vi "Read Configuration.vi"(0 "Config File Path":path, 5 "Scalar Or Vector":string="Scalar", 9 "Fixture Or Cal":string="Fixture", 11 "Error in (no error)":errorcluster) -> (4 "Path Groups out":refnum<class "Path Group.lvclass">[](array[class]), 6 "Path Count":i32, 15 "Error out":errorcluster)   [LabVIEW 2023, in "RFCalAndFixtureCharact.Common.lvlib"]
uses:
  RFCalAndFixtureCharact.Common.lvlib
  Base Classes/Path Group/Path Group.lvclass
  <vilib>/Utility/file.llb/Read Delimited Spreadsheet (string).vi
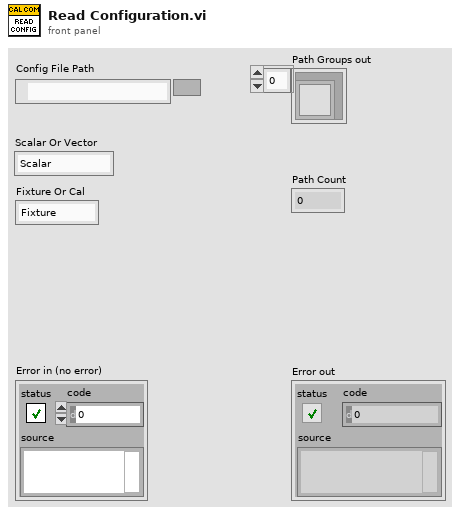
[diagram p1: front panel]
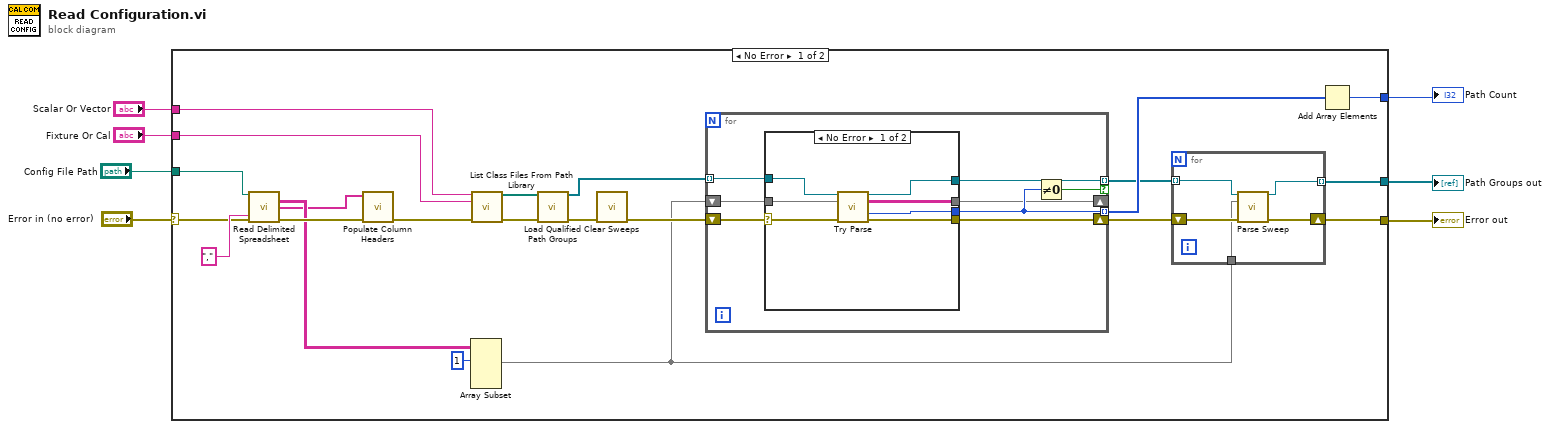
[diagram p0: block diagram]
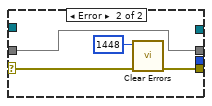
[diagram p2: hidden frame]
diagram:
  n1 = case shown="No Error" "Error in (no error)" {
    selector: "Error in (no error)" -> [w20 w54]
    tunnel: [w8 w54] -> w6
    tunnel: [w27 _] -> w5
    tunnel: "Config File Path" -> [w21 _]
    tunnel: [w10 _] -> w3
    tunnel: "Fixture Or Cal" -> [w17 _]
    tunnel: "Scalar Or Vector" -> [w16 _]
    frame No Error {
      n2 = call-poly <vilib>:"Read Delimited Spreadsheet.vi"("file path (dialog if empty)"=w21, "error in (no error)"=w20, "delimiter (\\t)"="," ("delimiter (\\t)")) -> ("all rows"=w24:string[][], "first row"=w22:string[], "error out"=w25:errorcluster)  [unwired: 7 in, 3 out]
      n3 = call "Populate Column Headers.vi"("error in (no error)"=w25, "Column Headers"=w22) -> ("error out"=w15:errorcluster)  [unwired: 9 in]
      n4 = Array Subset(array=w24, index (row)=1 ("index")) -> (w9:string[][])  [unwired: 3 in]
      n5 = call "List Class Files From Path Library.vi"("Specified Folder Name"=w16, "Fixture Or Cal"=w17, "Error in"=w15) -> ("Class Files"=w18:path[], "Error out"=w19:errorcluster)  [unwired: 11 in]
      n6 = call "Load Qualified Path Groups.vi"("Class Files"=w18, "error in"=w19) -> ("Path Groups out"=w29:refnum<class "Path Group.lvclass">[], "error out"=w14:errorcluster)  [unwired: 12 in]
      n7 = call "Clear Sweeps.vi"("error in (no error)"=w14) -> ("error out"=w13:errorcluster)  [unwired: 14 in]
      n8 = for {
        tunnel: w29 -> [w36] mode=indexing
        tunnel: [w37] -> w28 mode=indexing
        shift-right: [w40] -> w11
        shift-left: w13 -> [w42]
        tunnel: [w39] -> w12 mode=indexing if=w38
        shift-right: [w35] -> _
        shift-left: w9 -> [w41]
        n9 = case shown="No Error" w42 {
          selector: w42 -> [w45 w53]
          tunnel: w36 -> [w46 _]
          tunnel: w41 -> [w49 w50]
          tunnel: [w48 w52] -> w40
          tunnel: [w44 _] -> w37
          tunnel: [w47 _] -> w39
          tunnel: [w43 w50] -> w35
          frame No Error {
            n10 = call-dynamic "Try Parse.vi"("Path Group in"=w46, "Config Rows"=w49, "error in (no error)"=w45) -> ("Path Group out"=w47:refnum<class "Path Group.lvclass">, "Unparsed Rows"=w43:string[][], "Path Count"=w44:i32, "error out"=w48:errorcluster)  [unwired: 9 in]
          }
          frame Error {
            n11 = call <vilib>:"Clear Errors.vi"("error in (no error)"=w53, "specific error code to clear (0: all)"=1448) -> ("error out"=w52:errorcluster)  [unwired: 4 in, 1 out]
          }
        }
        n12 = Not Equal To 0?(x=w37) -> (x != 0?=w38:bool)
      }
      n13 = for {
        tunnel: w12 -> [w32] mode=indexing
        shift-right: [w33] -> w8
        shift-left: w11 -> [w34]
        tunnel: [w31] -> w10 mode=indexing
        tunnel: w9 -> [w30]
        n14 = call "Parse Sweep.vi"("Path Group in"=w32, "Config Rows"=w30, "error in (no error)"=w34) -> ("Path Group out"=w31:refnum<class "Path Group.lvclass">, "error out"=w33:errorcluster)  [unwired: 11 in]
      }
      n15 = Add Array Elements(numeric array=w28) -> (sum=w27:i32)
    }
    frame Error {
    }
  }
  "Error out" <- w6
  "Path Count" <- w5
  "Path Groups out" <- w3
